vi "Initialize Library Path.vi"(11 "library path":path) -> (0 "error out":errorcluster, 2 "modules found":i32)   [LabVIEW 2020, in "AIM ARINC 429 Hardware API.lvlib"]
uses:
  AIM ARINC 429 Hardware API.lvlib
  <instrlib>/_AIM 429/GlobalDLLPath.vi
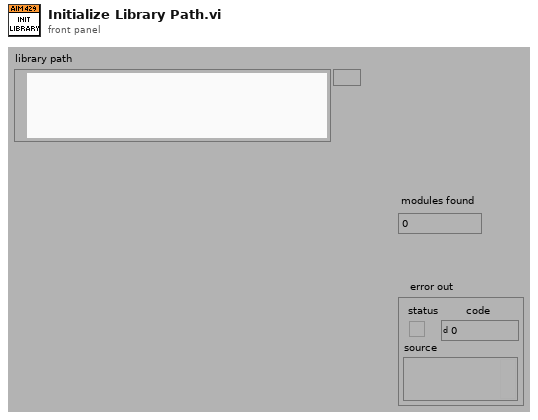
[diagram p1: front panel]
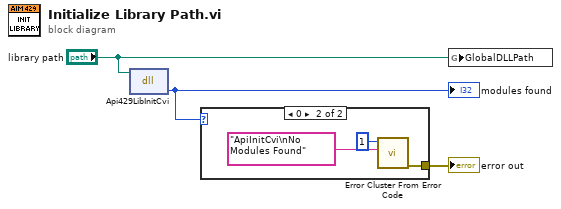
[diagram p0: block diagram]
diagram:
  n1 = dll-call lib="api_civ.9.dll" fn="Api429LibInitCvi"(path in="library path") -> ("modules found"=w2:i32)  [unwired: 2 in, 2 out]
  "modules found" <- w2
  n2 = case shown="0" w2 {
    tunnel: [_ w6] -> w3
    frame Default {
    }
    frame 0 {
      n3 = call <vilib>:"Error Cluster From Error Code.vi"("error message (\"\")"="ApiInitCvi\nNo Modules Found", "error code (0)"=1) -> ("error out"=w6:errorcluster)  [unwired: 7 in]
    }
  }
  "error out" <- w3
  n4 = global write "GlobalDLLPath.vi" "GlobalDLLPath"("library path") -> ()
